vi "Parse Object.vi"(8 "error in (no error)":errorcluster, 10 "Index In":i32, 11 "JSON String":string) -> (0 "error out":errorcluster, 2 "Index Out":i32, 3 "JSON Value out":refnum<class "JSON Value.lvclass">)   [LabVIEW 2016, in "JSON Value.lvclass"]
uses:
  JSON Value.lvclass
  subVIs/Errors.ctl
  subVIs/Token Type.ctl
  New JSON Value/New JSON ({Value[]}).vi
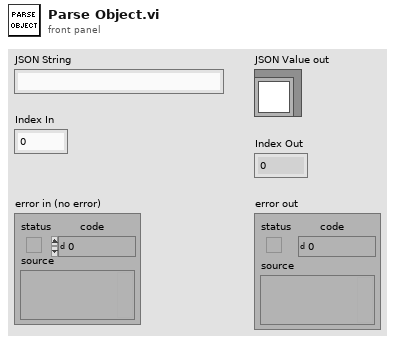
[diagram p1: front panel]
types:
  T1 = typedef "JSON Value.lvclass/Errors.ctl" = enum16{"No key", "Key path type", "Array OOB", "Type Mismatch", "Invalid Token"}
  T2 = typedef "JSON Value.lvclass/Token Type.ctl" = enum16{"NONE", "CURLY_OPEN", "CURLY_CLOSE", "SQUARED_OPEN", "SQUARED_CLOSE", "COLON", "COMMA", "STRING", "NUMBER", "TRUE", "FALSE", "NULL"}
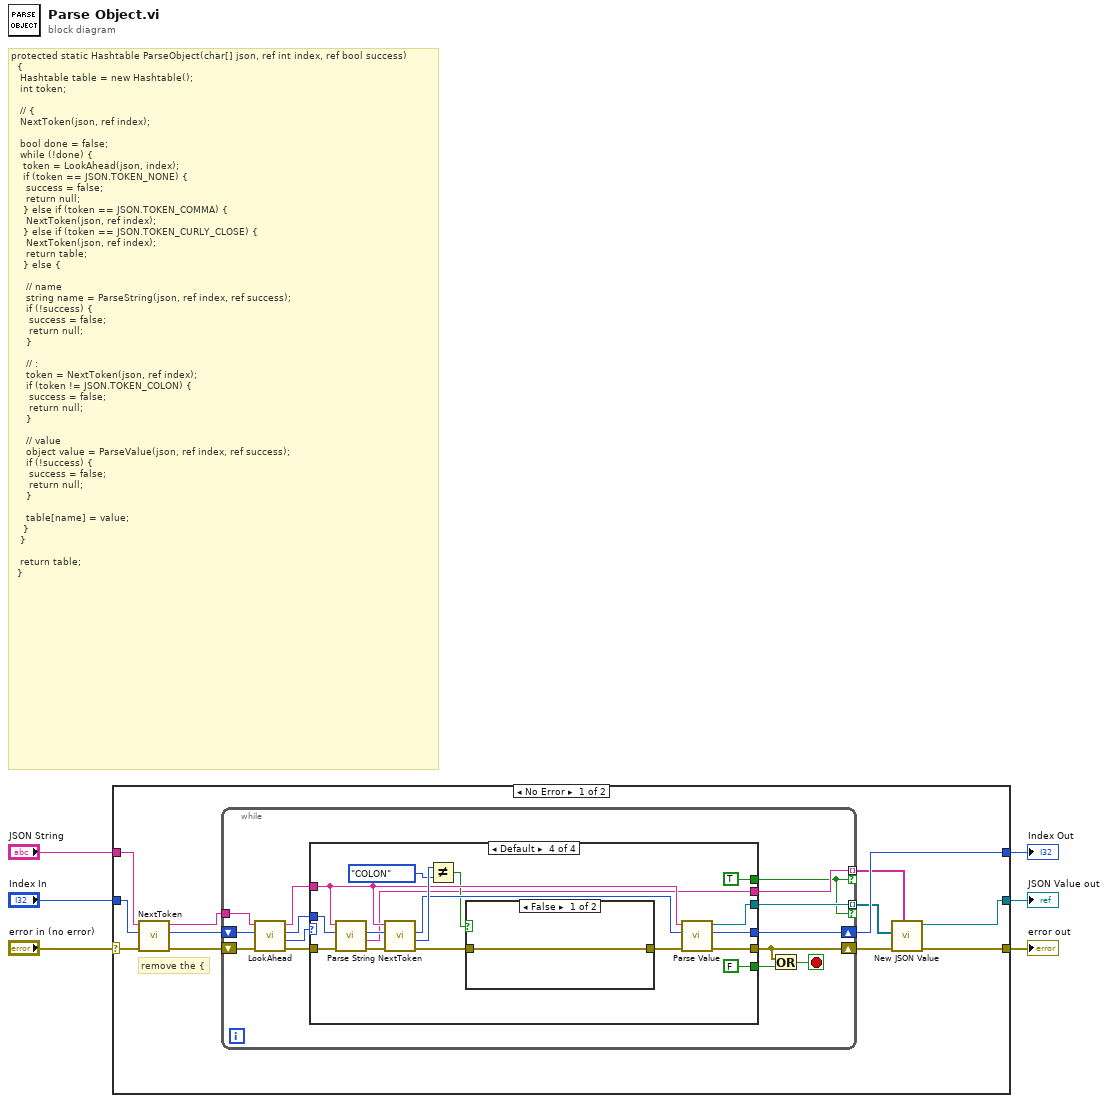
[diagram p0: block diagram]
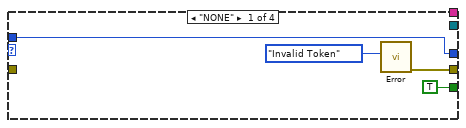
[diagram p2: hidden frame]
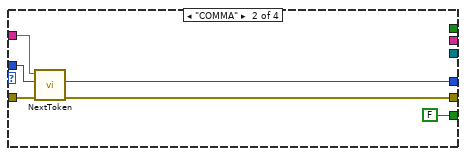
[diagram p3: hidden frame]
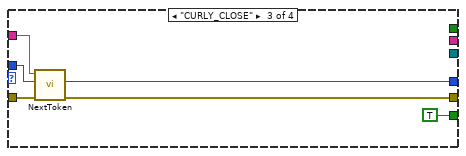
[diagram p4: hidden frame]
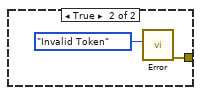
[diagram p5: hidden frame]
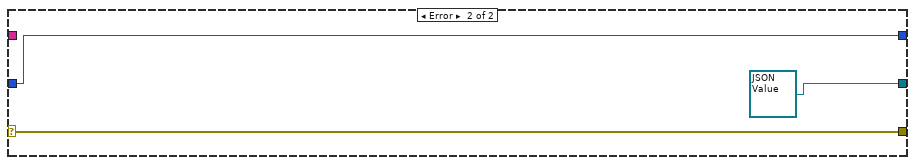
[diagram p6: hidden frame]
diagram:
  # "protected static Hashtable ParseObject(char[] json, ref int index, ref bool success)\n\t\t{\n\t\t\tHashtable table = new Hashtable();\n\t\t\tint token;\n\n\t\t\t// {\n\t\t\tNextToken(json, ref index);\n\n\t\t\tbool done = false;\n\t\t\twhile (!done) {\n\t\t\t\ttoken = LookAhead(json, index);\n\t\t\t\tif (token == JSON.TOKEN_NONE) {\n\t\t\t\t\tsuccess = false;\n\t\t\t\t\treturn null;\n\t\t\t\t} else if (token == JSON.TOKEN_COMMA) {\n\t\t\t\t\tNextToken(json, ref index);\n\t\t\t\t} else if (token == JSON.TOKEN_CURLY_CLOSE) {\n\t\t\t\t\tNextToken(json, ref index);\n\t\t\t\t\treturn table;\n\t\t\t\t} else {\n\n\t\t\t\t\t// name\n\t\t\t\t\tstring name = ParseString(json, ref index, ref success);\n\t\t\t\t\tif (!success) {\n\t\t\t\t\t\tsuccess = false;\n\t\t\t\t\t\treturn null;\n\t\t\t\t\t}\n\n\t\t\t\t\t// :\n\t\t\t\t\ttoken = NextToken(json, ref index);\n\t\t\t\t\tif (token != JSON.TOKEN_COLON) {\n\t\t\t\t\t\tsuccess = false;\n\t\t\t\t\t\treturn null;\n\t\t\t\t\t}\n\n\t\t\t\t\t// value\n\t\t\t\t\tobject value = ParseValue(json, ref index, ref success);\n\t\t\t\t\tif (!success) {\n\t\t\t\t\t\tsuccess = false;\n\t\t\t\t\t\treturn null;\n\t\t\t\t\t}\n\n\t\t\t\t\ttable[name] = value;\n\t\t\t\t}\n\t\t\t}\n\n\t\t\treturn table;\n\t\t}"
  n1 = case shown="No Error" "error in (no error)" {
    selector: "error in (no error)" -> [w14 w70]
    tunnel: [w7 w70] -> w5
    tunnel: "Index In" -> [w15 w71]
    tunnel: [w18 w71] -> w3
    tunnel: [w9 refnum<class "JSON Value.lvclass"> refnum ("JSON Object in")] -> w1
    tunnel: "JSON String" -> [w12 _]
    frame No Error {
      # "remove the {"
      n2 = call "NextToken.vi"("error in (no error)"=w14, "Index In"=w15, "JSON String"=w12) -> ("error out"=w17:errorcluster, "Index Out"=w16:i32, "JSON String Passthrough"=w13:string)  [unwired: 5 in, 1 out]
      n3 = while {
        tunnel: w13 -> [w31]
        shift-right: [w26] -> w18
        shift-left: w16 -> [w30]
        shift-right: [w22] -> w8
        shift-left: w17 -> [w32]
        tunnel: [w21] -> w11 mode=indexing if=w19
        tunnel: [w20] -> w10 mode=indexing if=w19
        stop <- w23 stop-if-true
        n4 = call "LookAhead.vi"("error in (no error)"=w32, "Index"=w30, "JSON String"=w31) -> ("error out"=w28:errorcluster, "TOKEN"=w29:T2, "Index Passthrough"=w27:i32, "JSON String Passthrough"=w25:string)  [unwired: 5 in]
        n5 = case shown="Default" w29 {
          tunnel: [TRUE FALSE TRUE FALSE] -> w24
          tunnel: w28 -> [_ w42 w48 w65]
          tunnel: [w34 w39 w45 w56] -> w22
          tunnel: w27 -> [w35 w41 w47 w64]
          tunnel: [w35 w40 w46 w57] -> w26
          tunnel: w25 -> [_ w37 w43 w59]
          tunnel: [_ _ _ w51] -> w21
          tunnel: [_ _ _ w50] -> w20
          tunnel: [_ _ _ TRUE] -> w19
          frame "NONE" {
            n6 = call "Error.vi"(9:Errors."Invalid Token") -> ("error out"=w34:errorcluster)  [unwired: 9 in]
          }
          frame "COMMA" {
            n7 = call "NextToken.vi"("error in (no error)"=w42, "Index In"=w41, "JSON String"=w37) -> ("error out"=w39:errorcluster, "Index Out"=w40:i32)  [unwired: 5 in, 2 out]
          }
          frame "CURLY_CLOSE" {
            n8 = call "NextToken.vi"("error in (no error)"=w48, "Index In"=w47, "JSON String"=w43) -> ("error out"=w45:errorcluster, "Index Out"=w46:i32)  [unwired: 5 in, 2 out]
          }
          frame Default {
            n9 = call "Parse String.vi"("error in (no error)"=w65, "Index In"=w64, "JSON String"=w59) -> ("error out"=w63:errorcluster, "Parsed String"=w51:string, "Index Out"=w62:i32)  [unwired: 5 in, 1 out]
            n10 = call "NextToken.vi"("error in (no error)"=w63, "Index In"=w62, "JSON String"=w59) -> ("error out"=w52:errorcluster, "TOKEN"=w61:T2, "Index Out"=w58:i32)  [unwired: 5 in, 1 out]
            n11 = Not Equal?(x=w61, y=Token_Type."COLON") -> (x != y?=w54:bool)
            n12 = case shown="False" w54 {
              tunnel: [w66 w67] -> w53
              tunnel: w52 -> [w66 _]
              frame False {
              }
              frame True {
                n13 = call "Error.vi"(9:Errors."Invalid Token") -> ("error out"=w67:errorcluster)  [unwired: 9 in]
              }
            }
            n14 = call "Parse Value.vi"("error in (no error)"=w53, "Index In"=w58, "JSON String"=w59) -> ("error out"=w56:errorcluster, "Index Out"=w57:i32, "JSON Value out"=w50:refnum<class "JSON Value.lvclass">)  [unwired: 6 in]
          }
        }
        n15 = Or(x=w22, y=w24) -> (x .or. y?=w23:bool)
      }
      n16 = call-poly "New JSON Value.vi"("keys"=w11, "error in (no error)"=w8, "values"=w10) -> ("error out"=w7:errorcluster, "JSON Value out"=w9:refnum<class "JSON Value.lvclass">)  [unwired: 7 in]
    }
    frame Error {
    }
  }
  "error out" <- w5
  "Index Out" <- w3
  "JSON Value out" <- w1
